vi "Update_CMD_Build.vi"(4 "RFID":string, 5 "Machine No":i32=2, 8 "error in (no error)":errorcluster, 9 "Variant":variant) -> (2 "error out":errorcluster, 3 "Update Query":string)   [LabVIEW 2020]
uses:
  MS SQL/MS_Global.vi
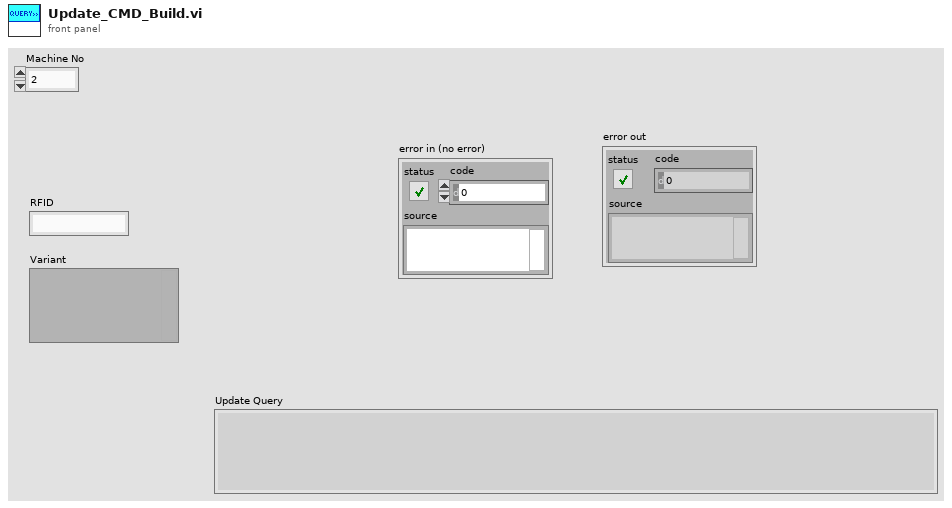
[diagram p1: front panel]
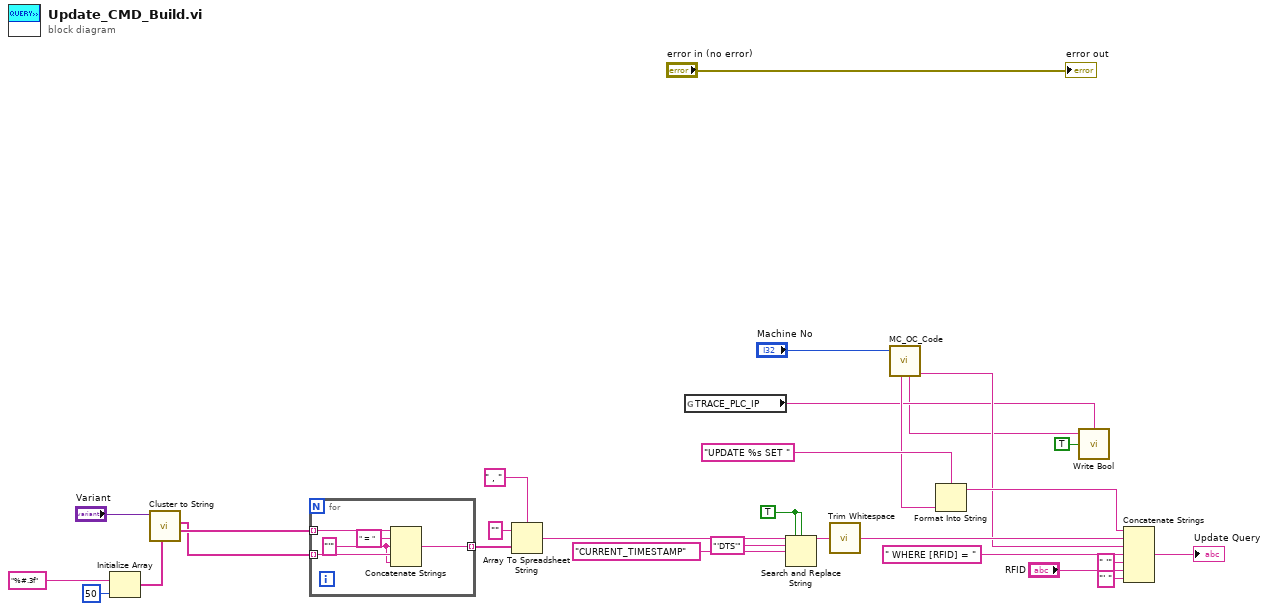
[diagram p0: block diagram]
diagram:
  w19 = TRUE ("replace all? (F)")
  n1 = Initialize Array("%#.3f" ("delimiter (Tab)"), 50 ("dimension size")) -> (w7:string[])
  n2 = call <userlib>:"Cluster to String.vi"("Format IN"=w7, "Variant In"="Variant") -> ("Format String Name"=w2:string[], "Format String Array"=w1:string[])  [unwired: 6 in, 2 out]
  n3 = for {
    tunnel: w1 -> [w34] mode=indexing
    tunnel: [w32] -> w18 mode=indexing
    tunnel: w2 -> [w31] mode=indexing
    w33 = "'" ("string")
    n4 = Concatenate Strings(w31, " = " ("string"), w33, w34, w33) -> (w32:string)
  }
  n5 = Array To Spreadsheet String(delimiter (Tab)=" , ", array=w18, 3:"" ("format string")) -> (spreadsheet string=w22:string)
  n6 = global read "MS_Global.vi" "TRACE_PLC_IP"() -> (w5:string)
  n7 = Search and Replace String(replace all?=w19, case sensitive?=w19, input string=w22, search string="'DTS'", replace string="CURRENT_TIMESTAMP" ("DTS_SCAN")) -> (result string=w24:string)  [unwired: 3 in, 3 out]
  n8 = call <vilib>:"Trim Whitespace.vi"("string"=w24) -> ("trimmed string"=w13:string)  [unwired: 1 in]
  n9 = call "MC_OC_Code.vi"("index"="Machine No") -> ("Code Query"=w11:string, "Data Saved Tag"=w4:string, "Table Name"=w10:string)  [unwired: 4 in, 4 out]
  n10 = Format Into String(format string="UPDATE %s SET " ("Table Name 2"), w10) -> (resulting string=w14:string)  [unwired: 2 in, 1 out]
  n11 = call "Write Bool.vi"("Network Path"=w5, "Int"=TRUE, "Tag Name"=w4) -> ()  [unwired: 2 in]
  n12 = Concatenate Strings(w14, w13, w11, " WHERE [RFID] = " ("Query"), " '" ("string"), "RFID", "' " ("string")) -> (→"Update Query":string)
  "error out" <- "error in (no error)"
